vi "Task Type Change.vi"(8 "error in (no error)":errorcluster, 11 "GUI in":refnum<class "GUI.lvclass">) -> (0 "error out":errorcluster, 3 "GUI out":refnum<class "GUI.lvclass">)   [LabVIEW 2020, in "GUI.lvlib" / "GUI.lvclass"]
uses:
  GUI.lvclass
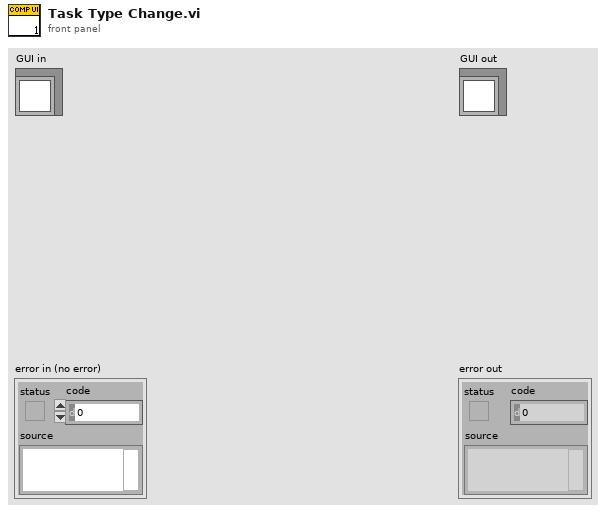
[diagram p1: front panel]
types:
  T1 = typedef "Automate df.ctl" = cluster{"Automate?":bool, "Num Parabs":u16, "Patterns Array":u8[][], "Phase Array":i32[][]}
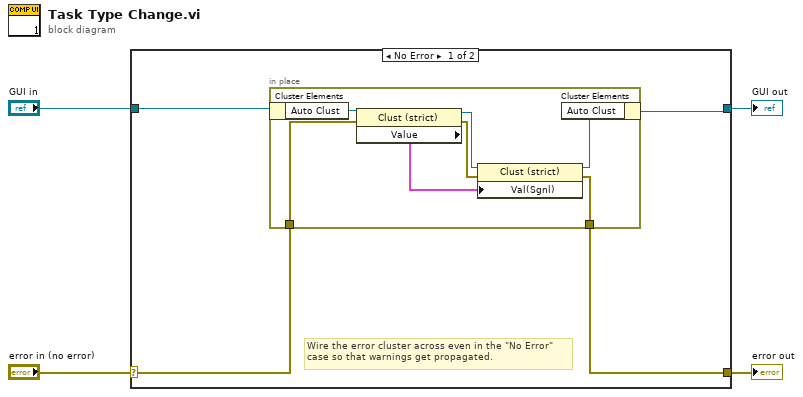
[diagram p0: block diagram]
diagram:
  n1 = case shown="No Error" "error in (no error)" {
    selector: "error in (no error)" -> [w6 w17]
    tunnel: [w5 w17] -> w3
    tunnel: [w7 w16] -> w1
    tunnel: "GUI in" -> [w8 w16]
    frame No Error {
      # "Wire the error cluster across even in the \"No Error\"\ncase so that warnings get propagated."
      n2 = in-place {
        in-place-border: w6 -> [w14]
        in-place-border: [w9] -> w5
        n3 = in-place-cluster #1(w8) -> ("Auto Clust"=w15:refnum<vi>)
        n4 = property class="Clust (strict)"(reference=w15, error in=w14) -> (reference out=w13:refnum<vi>, error out=w12:errorcluster, "Value"=w11:T1)
        n5 = property class="Clust (strict)"(reference=w13, error in=w12, "Val(Sgnl)"=w11) -> (reference out=w10:refnum<vi>, error out=w9:errorcluster)
        n6 = in-place-cluster #1("Auto Clust"=w10) -> (w7:refnum<class "GUI.lvclass">)
      }
    }
    frame Error {
    }
  }
  "error out" <- w3
  "GUI out" <- w1
